vi "Get Segments in Range.vi"(8 "error in (no error)":errorcluster, 10 "Time Range":T3, 11 "Waveform Buffer in":refnum<class "Waveform Buffer.lvclass">) -> (0 "error out":errorcluster, 1 "dt":dbl, 2 "Wfm Segments":T1[](array[typedef]), 3 "Waveform Buffer out":refnum<class "Waveform Buffer.lvclass">, 4 "tf Modified?":bool[](array[boolean]))   [LabVIEW 2015, in "Waveform Buffer.lvclass"]
uses:
  Waveform Buffer.lvclass
  Time Range.ctl
  Wfm Segment.ctl
  Data Point.ctl
  Waveform Buffer.lvclass/Waveform Buffer.ctl
  Shift Point by Samples.vi
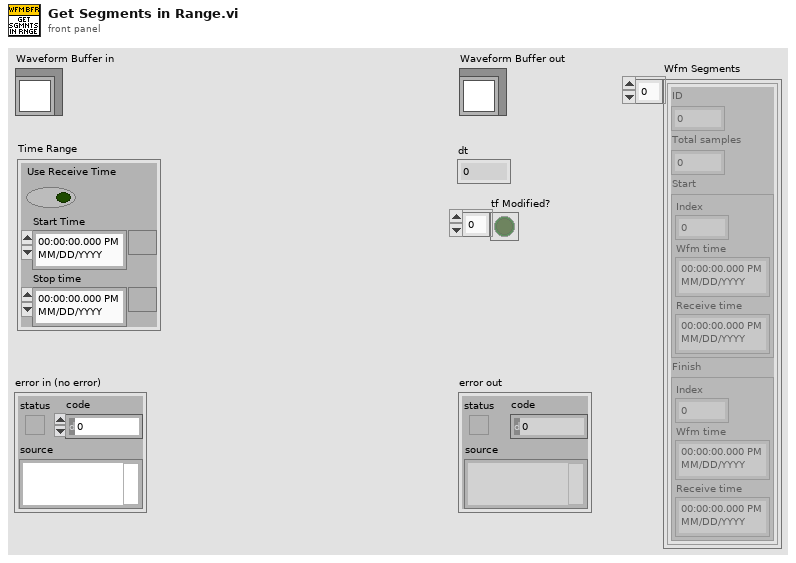
[diagram p1: front panel]
types:
  T1 = typedef "Waveform Buffer.lvclass/Wfm Segment.ctl" = cluster{"ID":u64, "Total samples":i32, "Start":T2, "Finish":T2}
  T2 = typedef "Waveform Buffer.lvclass/Data Point.ctl" = cluster{"Index":i32, "Wfm time":timestamp, "Receive time":timestamp}
  T3 = typedef "Waveform Buffer.lvclass/Time Range.ctl" = cluster{"Use Receive Time":bool, "Start Time":timestamp, "Stop time":timestamp}
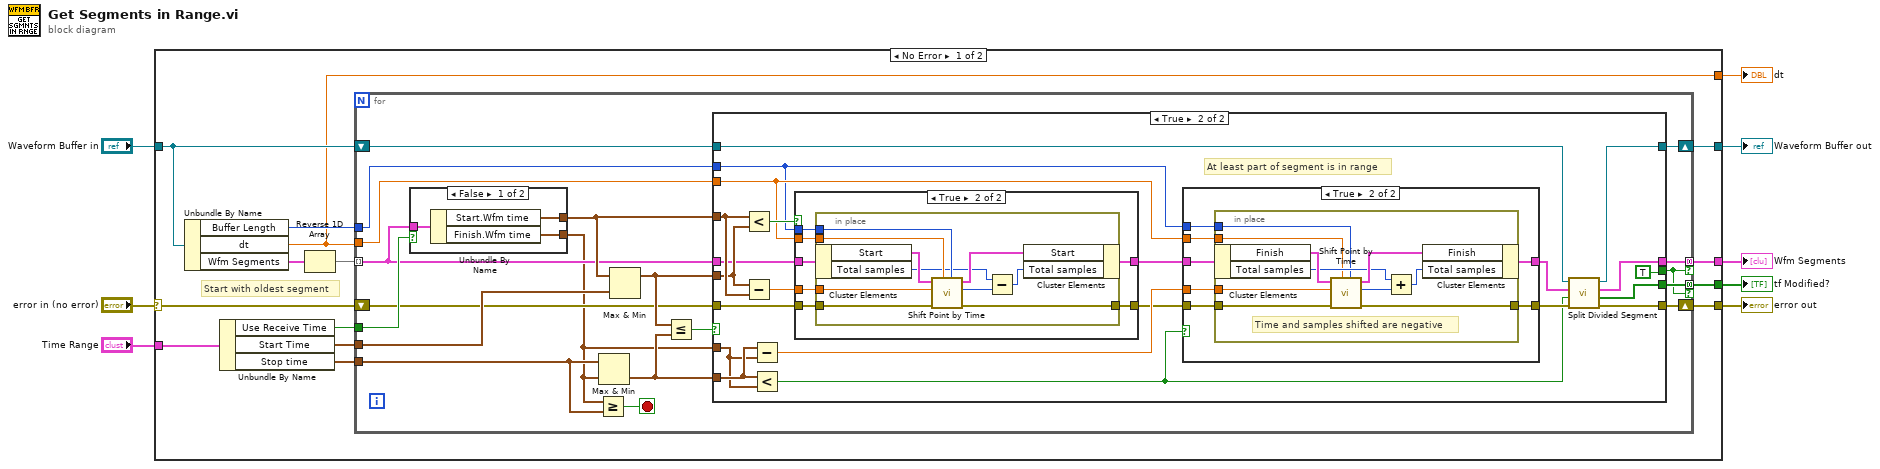
[diagram p0: block diagram]
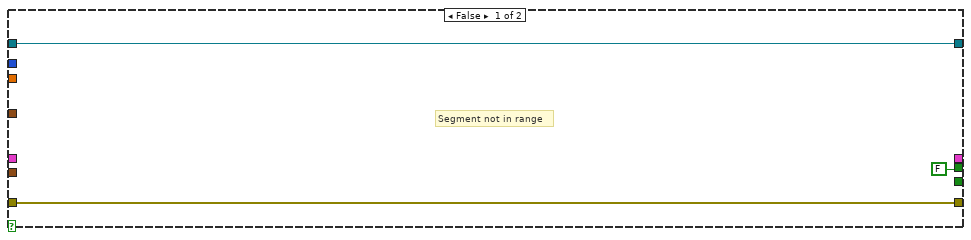
[diagram p2: hidden frame]
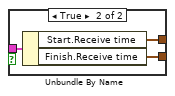
[diagram p5: hidden frame]
diagram:
  n1 = case shown="No Error" "error in (no error)" {
    selector: "error in (no error)" -> [w15 w112]
    tunnel: [w16 w112] -> w7
    tunnel: [w11 w111] -> w5
    tunnel: "Waveform Buffer in" -> [w12 w111]
    tunnel: "Time Range" -> [w22 _]
    tunnel: [w18 _] -> w3
    tunnel: [w10 _] -> w2
    tunnel: [w9 _] -> w1
    frame No Error {
      # "Start with oldest segment"
      n2 = Unbundle By Name(w12) -> ("Buffer Length"=w17:i32, "dt"=w10:dbl, "Wfm Segments"=w14:T1[])
      n3 = Unbundle By Name(w22) -> ("Use Receive Time"=w21:bool, "Start Time"=w20:timestamp, "Stop time"=w19:timestamp)
      n4 = Reverse 1D Array(array=w14) -> (reversed array=w13:T1[])
      n5 = for {
        tunnel: w21 -> [w41]
        tunnel: w20 -> [w40]
        tunnel: w19 -> [w27]
        tunnel: [w35] -> w18 mode=concatenating if=w23
        tunnel: w10 -> [w34]
        tunnel: w17 -> [w33]
        shift-right: [w32] -> w16
        shift-left: w15 -> [w31]
        tunnel: w13 -> [w30] mode=indexing
        shift-right: [w28] -> w11
        shift-left: w12 -> [w29]
        tunnel: [w24] -> w9 mode=concatenating if=w23
        stop <- w25 stop-if-true
        n6 = case shown="False" w41 {
          tunnel: w30 -> [w107 w110]
          tunnel: [w106 w109] -> w37
          tunnel: [w105 w108] -> w26
          frame False {
            n7 = Unbundle By Name(w107) -> ("Start.Wfm time"=w106:timestamp, "Finish.Wfm time"=w105:timestamp)
          }
          frame True {
            n8 = Unbundle By Name(w110) -> ("Start.Receive time"=w109:timestamp, "Finish.Receive time"=w108:timestamp)
          }
        }
        n9 = Greater Or Equal?(x=w26, y=w27) -> (x >= y?=w25:bool)
        n10 = Max & Min(x=w27, y=w26) -> (min(x,y)=w36:timestamp)  [unwired: 1 out]
        n11 = Max & Min(x=w37, y=w40) -> (max(x,y)=w38:timestamp)  [unwired: 1 out]
        n12 = Less Or Equal?(x=w38, y=w36) -> (x <= y?=w39:bool)
        n13 = case shown="True" w39 {
          tunnel: w38 -> [_ w63]
          tunnel: w37 -> [_ w64]
          tunnel: w36 -> [_ w61]
          tunnel: w26 -> [_ w60]
          tunnel: [FALSE TRUE] -> w23
          tunnel: w30 -> [_ w54]
          tunnel: [_ w49] -> w35
          tunnel: w34 -> [_ w58]
          tunnel: w33 -> [_ w57]
          tunnel: w31 -> [w44 w56]
          tunnel: [w44 w51] -> w32
          tunnel: w29 -> [w42 w48]
          tunnel: [w42 w47] -> w28
          tunnel: [_ w45] -> w24
          frame False {
            # "Segment not in range"
          }
          frame True {
            # "At least part of segment is in range"
            n14 = Less?(x=w64, y=w63) -> (x < y?=w66:bool)
            n15 = Subtract(x=w63, y=w64) -> (x-y=w62:dbl)
            n16 = Subtract(x=w61, y=w60) -> (x-y=w59:dbl)
            n17 = Less?(x=w61, y=w60) -> (x < y?=w46:bool)
            n18 = case shown="True" w66 {
              tunnel: w54 -> [w87 w91]
              tunnel: [w87 w90] -> w65
              tunnel: w62 -> [_ w94]
              tunnel: w58 -> [_ w93]
              tunnel: w57 -> [_ w92]
              tunnel: w56 -> [w86 w89]
              tunnel: [w86 w88] -> w55
              frame False {
                # "Start time is in range"
                # "start in range"
              }
              frame True {
                n19 = in-place {
                  in-place-border: w94 -> [w104]
                  in-place-border: w93 -> [w103]
                  in-place-border: w92 -> [w102]
                  in-place-border: w89 -> [w96]
                  in-place-border: [w95] -> w88
                  n20 = in-place-cluster #1(w91) -> ("Start"=w101:T2, "Total samples"=w98:i32)
                  n21 = call "Shift Point by Time.vi"("Buffer Length"=w102, "dt"=w103, "error in (no error)"=w96, "Time"=w104, "Data Point in"=w101) -> ("error out"=w95:errorcluster, "Samples shifted"=w99:i32, "Data Point out"=w100:T2)  [unwired: 4 in]
                  n22 = Subtract(x=w98, y=w99) -> (x-y=w97:i32)
                  n23 = in-place-cluster #1("Start"=w100, "Total samples"=w97) -> (w90:T1)
                }
              }
            }
            n24 = case shown="True" w46 {
              tunnel: w65 -> [w68 w74]
              tunnel: [w68 w73] -> w50
              tunnel: w59 -> [_ w75]
              tunnel: w58 -> [_ w72]
              tunnel: w57 -> [_ w71]
              tunnel: w55 -> [w67 w70]
              tunnel: [w67 w69] -> w52
              frame False {
                # "Finish time is in range"
              }
              frame True {
                n25 = in-place {
                  in-place-border: w75 -> [w85]
                  in-place-border: w72 -> [w79]
                  in-place-border: w71 -> [w78]
                  in-place-border: w70 -> [w77]
                  in-place-border: [w76] -> w69
                  # "Time and samples shifted are negative"
                  n26 = in-place-cluster #2(w74) -> ("Finish"=w83:T2, "Total samples"=w80:i32)
                  n27 = call "Shift Point by Time.vi"("Buffer Length"=w78, "dt"=w79, "error in (no error)"=w77, "Time"=w85, "Data Point in"=w83) -> ("error out"=w76:errorcluster, "Samples shifted"=w84:i32, "Data Point out"=w82:T2)  [unwired: 4 in]
                  n28 = Add(x=w80, y=w84) -> (x+y=w81:i32)
                  n29 = in-place-cluster #2("Finish"=w82, "Total samples"=w81) -> (w73:T1)
                }
              }
            }
            n30 = call "Split Divided Segment.vi"("error in (no error)"=w52, "tf Modified? in"=w46, "Wfm Segment in"=w50, "Waveform Buffer in"=w48) -> ("error out"=w51:errorcluster, "tf Modified? out"=w45:bool[], "Segments out"=w49:T1[], "Waveform Buffer out"=w47:refnum<class "Waveform Buffer.lvclass">)  [unwired: 4 in]
          }
        }
      }
    }
    frame Error {
    }
  }
  "error out" <- w7
  "Waveform Buffer out" <- w5
  "Wfm Segments" <- w3
  "dt" <- w2
  "tf Modified?" <- w1
